vi "OEE_SCREEN_2_OEE_into_cluster.vi"(6 "SCREEN_2":T2={"header_part_no"="-", "header_customer"="-", "performance_percentage"="-", "performance_target"="-", "performance_actual"="-", "performance_header"="PERFORMANCE", "performance_header_target"="TARGET", "performance_header_actual"="ACTUAL"}, 10 "config_info":string[](array[string]), 11 "SCREEN_1":T1={"header_date"="-", "header_time"="-", "header_takt"="-", "header_shift"="-", "OP10_actual"="-", "OP10_rejects"="-", "OP10_quality_yeild"="-", "OP10_pace"="-", "OP20_actual"="-", "OP20_rejects"="-", "OP20_quality_yeild"="-", "OP20_pace"="-", "OP30_actual"="-", "OP30_rejects"="-", "OP30_quality_yeild"="-", "OP30_pace"="-", "OP40_actual"="-", "OP40_rejects"="-", "OP40_quality_yeild"="-", "OP40_pace"="-", "OP50_actual"="-", "OP50_rejects"="-", "OP50_quality_yeild"="-", "OP50_pace"="-", "OP60_actual"="-", "OP60_rejects"="-", "OP60_quality_yeild"="-", "OP60_pace"="-", "OP70_actual"="-", "OP70_rejects"="-", "OP70_quality_yeild"="-", "OP70_pace"="-", "OP80_actual"="-", "OP80_rejects"="-", "OP80_quality_yeild"="-", "OP80_pace"="-", "OP90_actual"="-", "OP90_rejects"="-", "OP90_quality_yeild"="-", "OP90_pace"="-", "OP100_actual"="-", "OP100_rejects"="-", "OP100_quality_yeild"="-", "OP100_pace"="-", "OP110_actual"="-", "OP110_rejects"="-", "OP110_quality_yeild"="-", "OP110_pace"="-", "OP120_actual"="-", "OP120_rejects"="-", "OP120_quality_yeild"="-", "OP120_pace"="-", "OP130_actual"="-", "OP130_rejects"="-", "OP130_quality_yeild"="-", "OP130_pace"="-", "OP10_header"="OP10", "OP20_header"="OP20", "OP30_header"="OP30", "OP40_header"="OP40", "OP50_header"="OP50", "OP60_header"="OP60", "OP70_header"="OP70", "OP80_header"="OP80", "OP90_header"="OP90", "OP100_header"="OP100", "OP110_header"="OP110", "OP120_header"="OP120", "OP130_header"="OP130", "additional_info"="", "bottleneck_OP"="-", "bottleneck_header"="LINE BOTTLENECK"}) -> (4 "SCREEN_2":T2={"header_part_no"="-", "header_customer"="-", "performance_percentage"="-", "performance_target"="-", "performance_actual"="-", "performance_header"="PERFORMANCE", "performance_header_target"="TARGET", "performance_header_actual"="ACTUAL"})   [LabVIEW 2019]
uses:
  typedef/SCREEN_2.ctl
  SCREEN_1/typedef/SCREEN_1.ctl
panel:
  # "PERFORMANCE DATA OUTPUT BOARD #1"
  # "OP"
  # "Actual"
  # "Rejects"
  # "%FTTH"
  # "Pace"
  # "OP"
  # "Actual"
  # "Rejects"
  # "%FTTH"
  # "Pace"
  # "Performance Data Output Board #2"
  # "Performance Data Output Board #2"
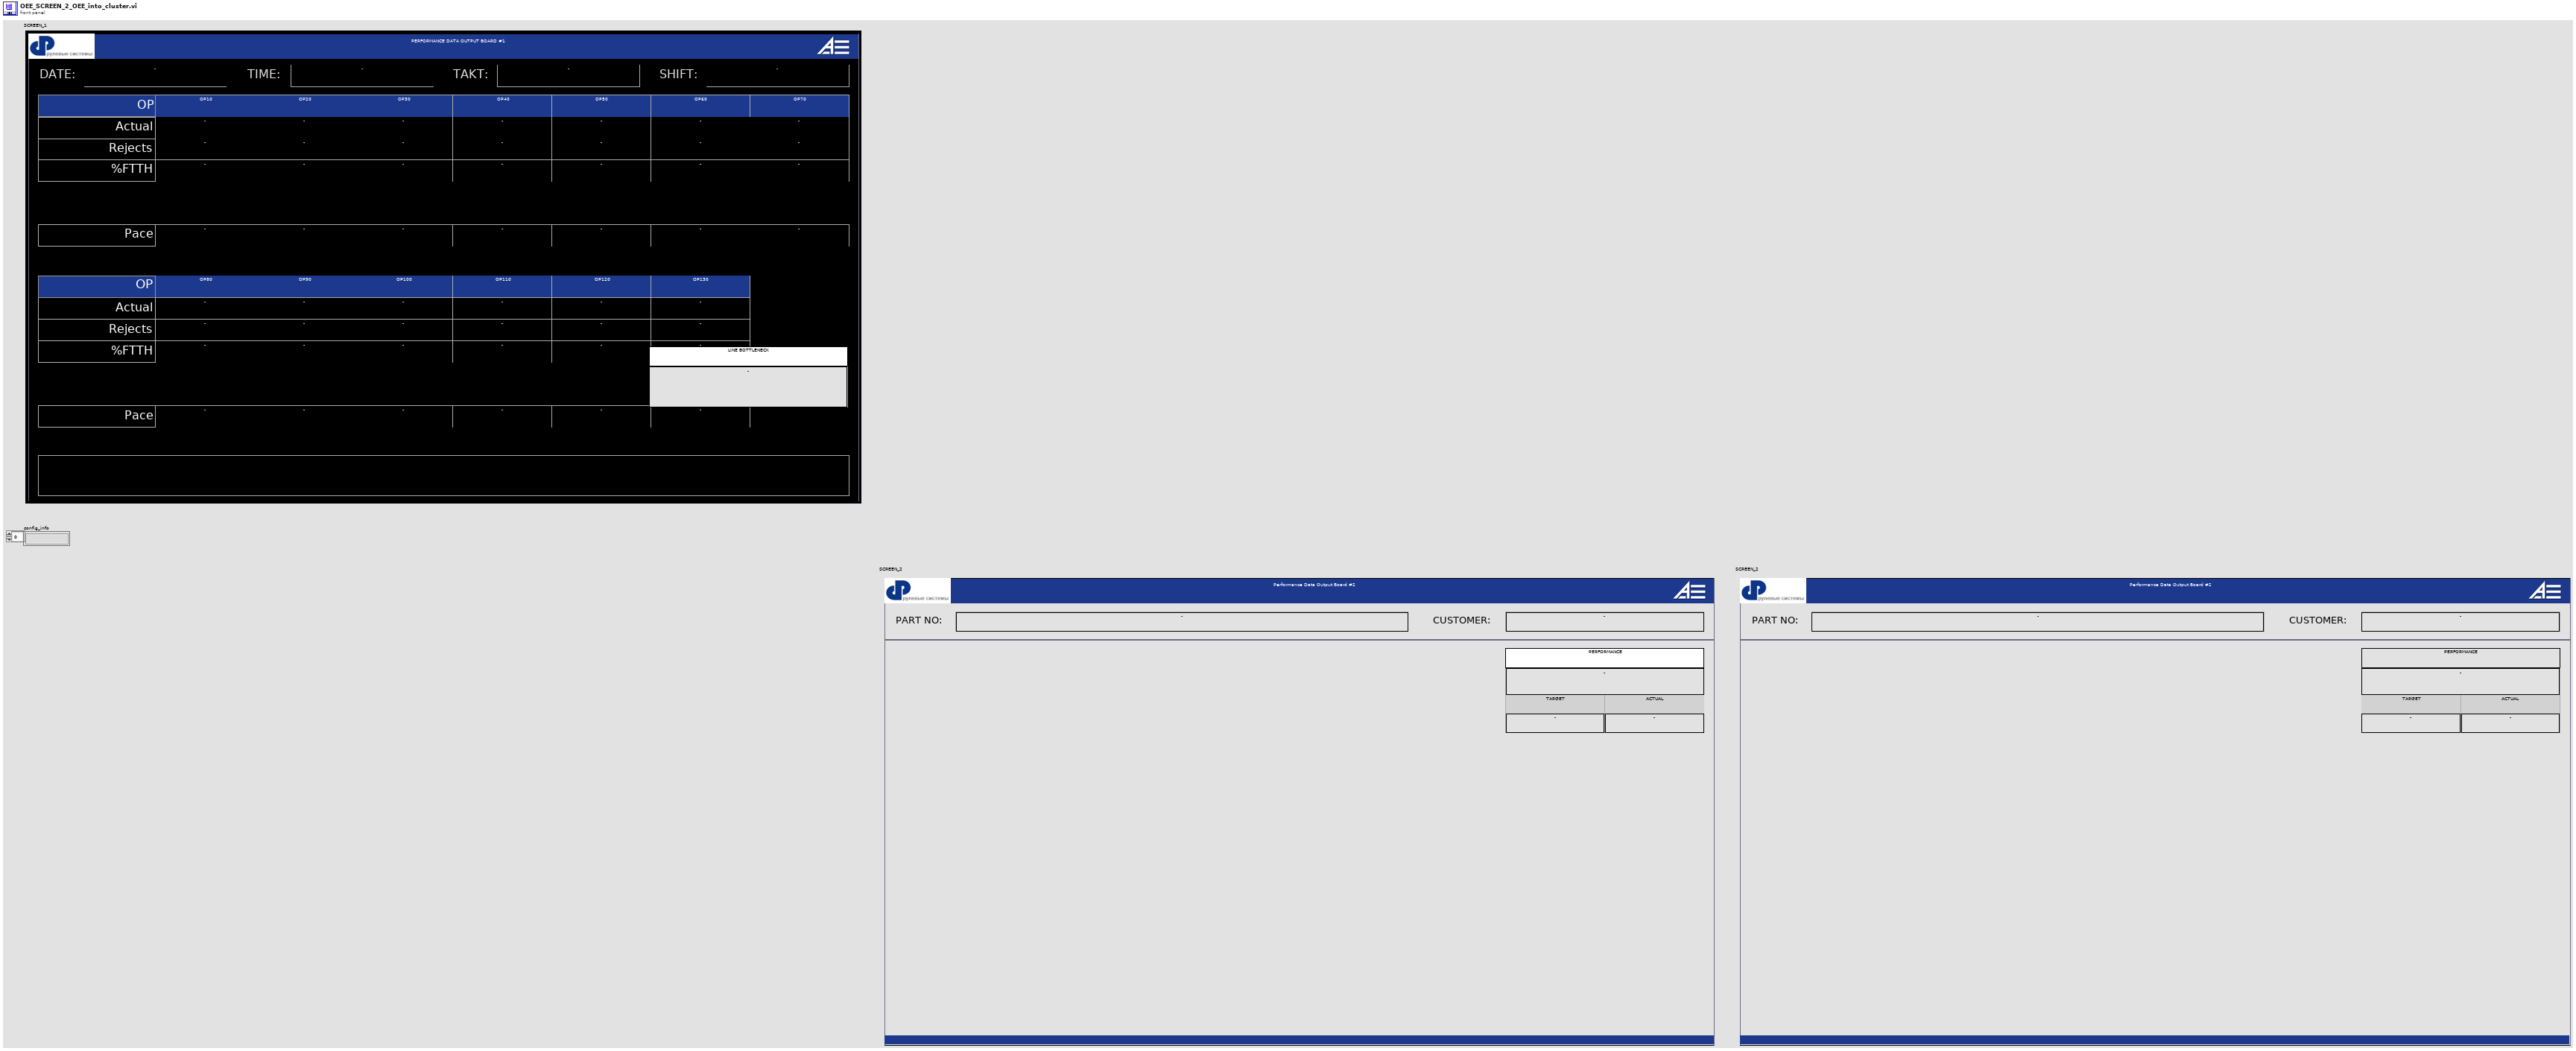
[diagram p1: front panel]
types:
  T1 = typedef "SCREEN_1.ctl" = cluster{"header_date":string, "header_time":string, "header_takt":string, "header_shift":string, "OP10_actual":string, "OP10_rejects":string, "OP10_quality_yeild":string, "OP10_pace":string, "OP20_actual":string, "OP20_rejects":string, "OP20_quality_yeild":string, "OP20_pace":string, "OP30_actual":string, "OP30_rejects":string, "OP30_quality_yeild":string, "OP30_pace":string, "OP40_actual":string, "OP40_rejects":string, "OP40_quality_yeild":string, "OP40_pace":string, "OP50_actual":string, "OP50_rejects":string, "OP50_quality_yeild":string, "OP50_pace":string, "OP60_actual":string, "OP60_rejects":string, "OP60_quality_yeild":string, "OP60_pace":string, "OP70_actual":string, "OP70_rejects":string, "OP70_quality_yeild":string, "OP70_pace":string, "OP80_actual":string, "OP80_rejects":string, "OP80_quality_yeild":string, "OP80_pace":string, "OP90_actual":string, "OP90_rejects":string, "OP90_quality_yeild":string, "OP90_pace":string, "OP100_actual":string, "OP100_rejects":string, "OP100_quality_yeild":string, "OP100_pace":string, "OP110_actual":string, "OP110_rejects":string, "OP110_quality_yeild":string, "OP110_pace":string, "OP120_actual":string, "OP120_rejects":string, "OP120_quality_yeild":string, "OP120_pace":string, "OP130_actual":string, "OP130_rejects":string, "OP130_quality_yeild":string, "OP130_pace":string, "OP10_header":string, "OP20_header":string, "OP30_header":string, "OP40_header":string, "OP50_header":string, "OP60_header":string, "OP70_header":string, "OP80_header":string, "OP90_header":string, "OP100_header":string, "OP110_header":string, "OP120_header":string, "OP130_header":string, "additional_info":string, "bottleneck_OP":string, "bottleneck_header":string}
  T2 = typedef "SCREEN_2.ctl" = cluster{"header_part_no":string, "header_customer":string, "performance_percentage":string, "performance_target":string, "performance_actual":string, "performance_header":string, "performance_header_target":string, "performance_header_actual":string}
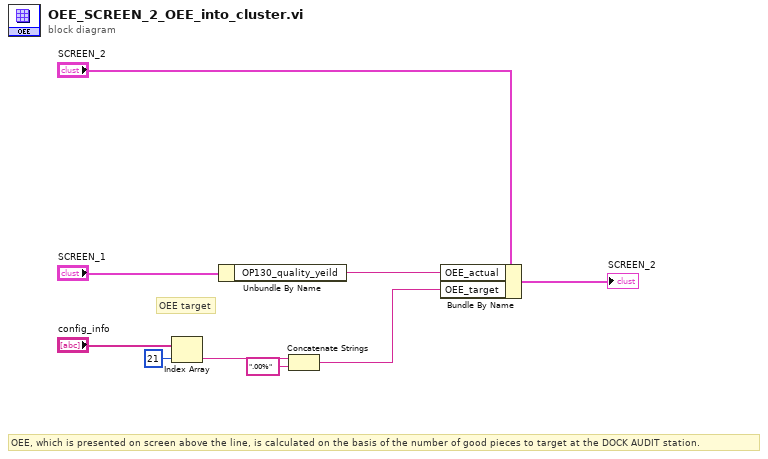
[diagram p0: block diagram]
diagram:
  # "OEE target"
  # "OEE, which is presented on screen above the line, is calculated on the basis of the number of good pieces to target at the DOCK AUDIT station."
  n1 = Index Array(array="config_info", index=21) -> (element=w3:string)
  n2 = Unbundle By Name("SCREEN_1") -> ("OP130_quality_yeild"=w4:string)
  n3 = Concatenate Strings(w3, ".00%" ("string")) -> (w2:string)
  n4 = Bundle By Name(cluster="SCREEN_2", "OEE_actual"=w4, "OEE_target"=w2) -> (→"SCREEN_2":T2)
